vi "Split.vi"(11 "String In":string) -> (2 "Splitted?":bool, 3 "String Out":string)   [LabVIEW 2021]
uses:
  <vilib>/regexp/Match Regular Expression.xnode
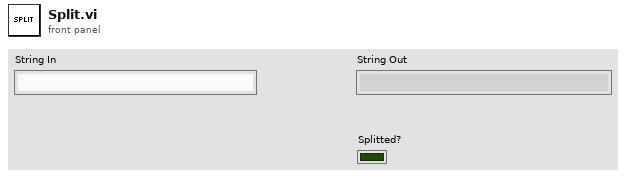
[diagram p1: front panel]
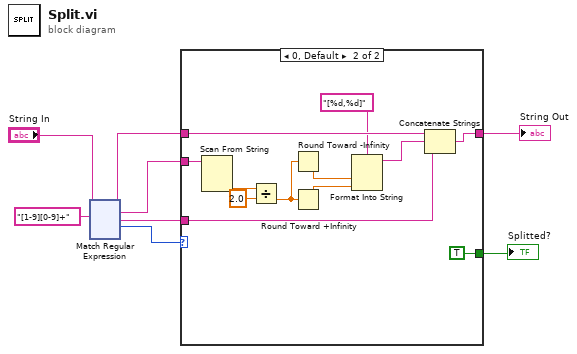
[diagram p0: block diagram]
diagram:
  n1 = xnode "Match Regular Expression"("input string"="String In", "regular expression"="[1-9][0-9]+") -> ("before match"=w6:string, "whole match"=w3:string, "after match"=w5:string, "offset past match"=w2:i32)  [unwired: 4 in, 1 out]
  n2 = case shown="0, Default" w2 {
    tunnel: w6 -> [w9 w21]
    tunnel: w5 -> [_ w20]
    tunnel: [w9 w19] -> w4
    tunnel: w3 -> [_ w18]
    tunnel: [_ TRUE] -> w1
    frame -1 {
    }
    frame 0, Default {
      n3 = Scan From String(input string=w18) -> (output 1=w17:dbl)  [unwired: 4 in, 3 out]
      n4 = Divide(x=w17, y=2.0) -> (x/y=w15:dbl)
      n5 = Round Toward -Infinity(1:w15) -> (0:w13:dbl)
      n6 = Round Toward +Infinity(x=w15) -> (ceil(x): smallest int >= x=w12:dbl)
      n7 = Format Into String(format string="[%d,%d]", w13, w12) -> (resulting string=w11:string)  [unwired: 2 in, 1 out]
      n8 = Concatenate Strings(w21, w11, w20) -> (w19:string)
    }
  }
  "String Out" <- w4
  "Splitted?" <- w1
